vi "Read Coils.vi"(8 "error in":errorcluster, 9 "number of inputs":u16, 10 "starting address":u16, 11 "Master CR in":refnum<class "Master CR.lvclass">) -> (0 "error out":errorcluster, 2 "coils":bool[](array[boolean]), 3 "Master CR out":refnum<class "Master CR.lvclass">)   [LabVIEW 2021, in "Master CR.lvclass"]
doc: "Reads <B>number of inputs</B> coils starting at <B>starting address</B> from the device."
uses:
  Master CR.lvclass
  Master CR.lvclass/Master CR.ctl
  Modbus_v121c/Data Model/Device Data Model.lvclass
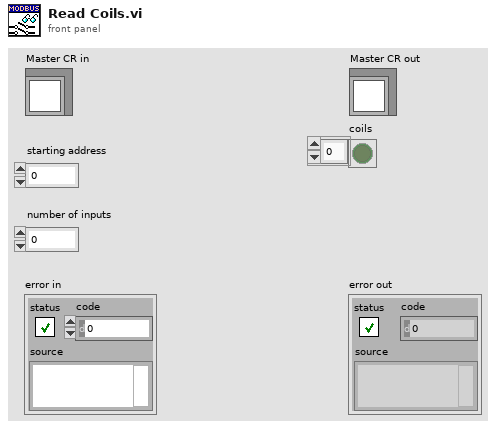
[diagram p1: front panel]
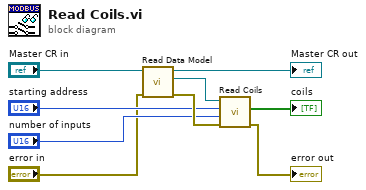
[diagram p0: block diagram]
diagram:
  n1 = call "Read Data Model.vi"("error in (no error)"="error in", "Master CR in"="Master CR in") -> ("error out"=w6:errorcluster, "Data Model"=w7:refnum<class "Device Data Model.lvclass">, "Master CR out"=→"Master CR out":refnum<class "Master CR.lvclass">)  [unwired: 7 in]
  n2 = call-dynamic "Read Coils.vi"("error in"=w6, "number of coils"="number of inputs", "starting address"="starting address", "device data model in"=w7) -> ("error out"=→"error out":errorcluster, "data"=→"coils":bool[])  [unwired: 5 in, 1 out]
